vi "Autonomous Independent-NewMode.vi"() -> ()   [LabVIEW 2016]
doc: "This VI is called when autonomous begins, and will automatically be terminated when autonomous ends. You can carry out timed or sensor driven robot movement independently without needing to return to the caller."
uses:
  <vilib>/Rock Robotics/WPI/ThirdParty/CanMotor/TalonSRX/WPI_CANTalonSRX_BrakeOverride.ctl
  <vilib>/Rock Robotics/WPI/Utilities/WPI_GetSetVariantRefNum.vi
  <vilib>/Rock Robotics/Network Tables/NT Write Numeric Array.vi
  <vilib>/Rock Robotics/Network Tables/NT Read String.vi
  <vilib>/Rock Robotics/Network Tables/NT Read Numeric Array.vi
  <vilib>/Rock Robotics/Network Tables/NT Read String Array.vi
  Robot Global Data.vi
  <vilib>/Rock Robotics/WPI/RobotDrive/WPI_RobotDriveMecanumDrive_Cartesian.vi
  <vilib>/addons/control/pid/pid.llb/PID (DBL).vi
  <vilib>/Rock Robotics/Network Tables/NT Write String.vi
  <vilib>/Rock Robotics/Network Tables/NT Write Number.vi
  <vilib>/addons/control/pid/NI_PID_pid.lvlib
  ADIS16448-Teensy/ADIS16448-Teensy.lvlib
  <vilib>/ptbypt/NI_PtbyPt.lvlib
panel:
  out "VisionError":dbl
  out "RotateError":dbl
  in  "VisionIterationDelay":i32=100
  in  "VisionSampleLength":i32=10
  in  "RotateIterationDelay":i32=100
  in  "RotateSampleLength":i32=30
  in  "ExitLimitVision":dbl=0.2
  in  "ExitLimitRotate":dbl=0.1
  in  "Vision Align PID Gains":cluster{"Kp":dbl, "Ki":dbl, "Kd":dbl, "Kf":dbl}={"Kp"=0.006, "Ki"=1.6e-05, "Kd"=0.0, "Kf"=0.0002} {"Kf" format="%.6f"; "Kd" format="%.6f"; "Ki" format="%.6f"; "Kp" format="%.6f"}
  in  "Rotate PID gains":cluster{"Kp":dbl, "Ki":dbl, "Kd":dbl, "Kf":dbl}={"Kp"=0.0048, "Ki"=3e-05, "Kd"=0.02048, "Kf"=0.0} {"Kf" format="%.6f"; "Kd" format="%.6f"; "Ki" format="%.8f"; "Kp" format="%.6f"}
  out "Rotate Chart":cluster{dbl, "Z Angle":dbl}(graph)
  in  "Drive Slow PID Values":T1={"proportional gain (Kc)"=0.01, "integral time (Ti, min)"=0.0, "derivative time (Td, min)"=0.001}
  in  "Drive Slow Limits":cluster{"output high":dbl, "output low":dbl}={"output high"=0.25, "output low"=-0.25}
  out "Drive Slow":cluster{dbl, "Z Angle":dbl}(graph)
  in  "Strafe Correction":dbl=0.05 step=0.05 format="%#_13g"
  in  "Strafe PID Values":T1={"proportional gain (Kc)"=0.2, "integral time (Ti, min)"=0.0, "derivative time (Td, min)"=0.003} {"proportional gain (Kc)" step=0.01; "integral time (Ti, min)" step=0.001; "derivative time (Td, min)" step=0.001}
  in  "Strafe Angle Limits":cluster{"output high":dbl, "output low":dbl}={"output high"=0.1, "output low"=-0.1}
  out "Strafe Chart":cluster{dbl, "Z Angle":dbl}(graph)
  out "Drive Fast":cluster{dbl, "Z Angle":dbl}(graph)
  in  "Drive Fast Limits":cluster{"output high":dbl, "output low":dbl}={"output high"=0.25, "output low"=-0.25}
  in  "Rotate outputs":cluster{"output high":dbl, "output low":dbl}={"output high"=1.0, "output low"=-1.0} {"output high" step=0.1; "output low" step=0.1}
  out "Vision Align Rotate Chart":cluster{dbl, "Z Angle":dbl}(graph)
  in  "Vision Align Limits":cluster{"output high":dbl, "output low":dbl}={"output high"=1.0, "output low"=-1.0} {"output high" step=0.1; "output low" step=0.1}
  in  "Drive Fast PID Values":T1={"proportional gain (Kc)"=0.01, "integral time (Ti, min)"=0.0, "derivative time (Td, min)"=0.001}
  # "NEW MODE"
  # "Marvin:\n.025\n0\n.001"
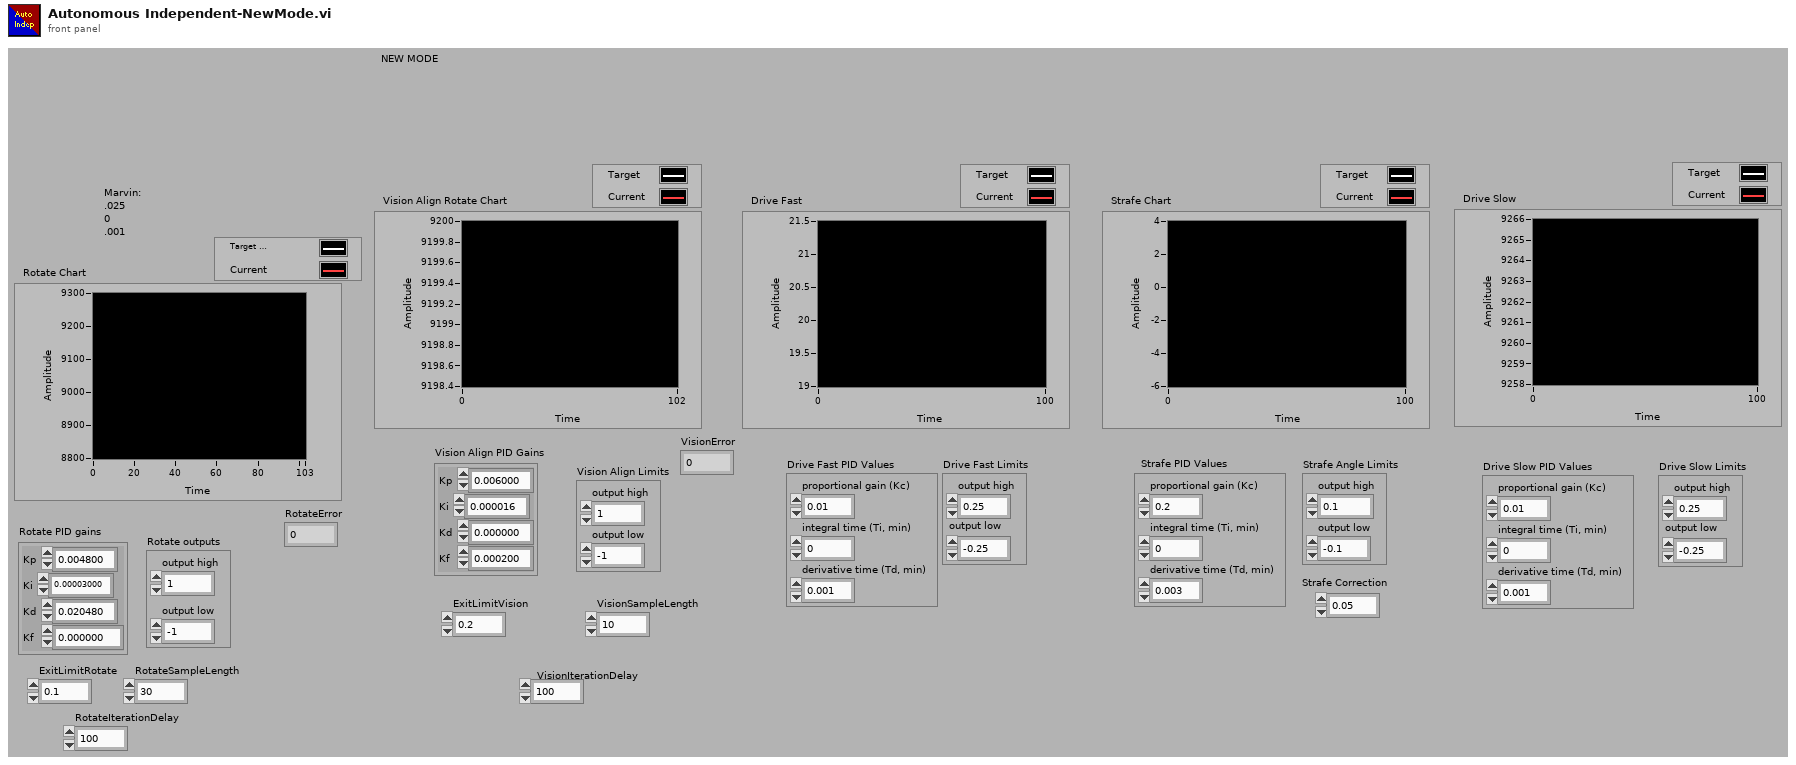
[diagram p1: front panel]
types:
  T1 = cluster{"proportional gain (Kc)":dbl, "integral time (Ti, min)":dbl, "derivative time (Td, min)":dbl}
  T2 = typedef "WPI_JoystickDevRef.ctl" = cluster{"Device":T3}
  T3 = typedef "WPI_JoystickDeviceEnum.ctl" = enum16{"USB 0", "USB 1", "USB 2", "USB 3", "USB 4", "USB 5"}
  T4 = typedef "WPI_CANTalonSRX_BrakeOverride.ctl" = enum8{"No Override", "Override to Coast", "Override to Brake"}
  T5 = typedef "WPI_MotorControlDeviceRef.ctl" = cluster{"DeviceStatus":errorcluster, "Type":T6, "PWM":cluster{"PWM Channel":T7, "DeadBand":T8}, "CAN":cluster{"Device Number":u8, "SetOutput VI Ref":variant, "GetOutput VI Ref":variant, "Enable VI Ref":variant, "Disable VI Ref":variant, "Data":variant}, "Invert":bool}
  T6 = typedef "WPI_MotorControlType.ctl" = enum16{"PWM", "CAN"}
  T7 = typedef "FPGA_DIOPWMChannel.ctl" = enum8{"PWM 0", "PWM 1", "PWM 2", "PWM 3", "PWM 4", "PWM 5", "PWM 6", "PWM 7", "PWM 8", "PWM 9", "PWM MXP 0", "PWM MXP 1", "PWM MXP 2", "PWM MXP 3", "PWM MXP 4", "PWM MXP 5", "PWM MXP 6", "PWM MXP 7", "PWM MXP 8", "PWM MXP 9", "Invalid"}
  T8 = typedef "WPI_PWMDeadband.ctl" = cluster{"Name":string, "maxPositivePwm":i32, "minPositivePwm":i32, "centerPwm":i32, "maxNegativePwm":i32, "minNegativePwm":i32, "angularRange":u16}
  T9 = typedef "WPI_SerialPortRef.ctl" = cluster{"DevStatus":errorcluster, "Serial Port Name":refnum<visa-resource-name>}
  T10 = typedef "WPI_RobotDriveDevRef.ctl" = cluster{"DevStatus":errorcluster, "Motors[]":T5[], "Square Inputs":bool, "Max Output":dbl}
  T11 = typedef "WPI_ServoDeviceRef.ctl" = cluster{"DeviceStatus":errorcluster, "PWM Channel":T7, "DeadBand":T8}
  T12 = cluster{"X Angle":dbl, "Y Angle":dbl, "Z Angle":dbl}
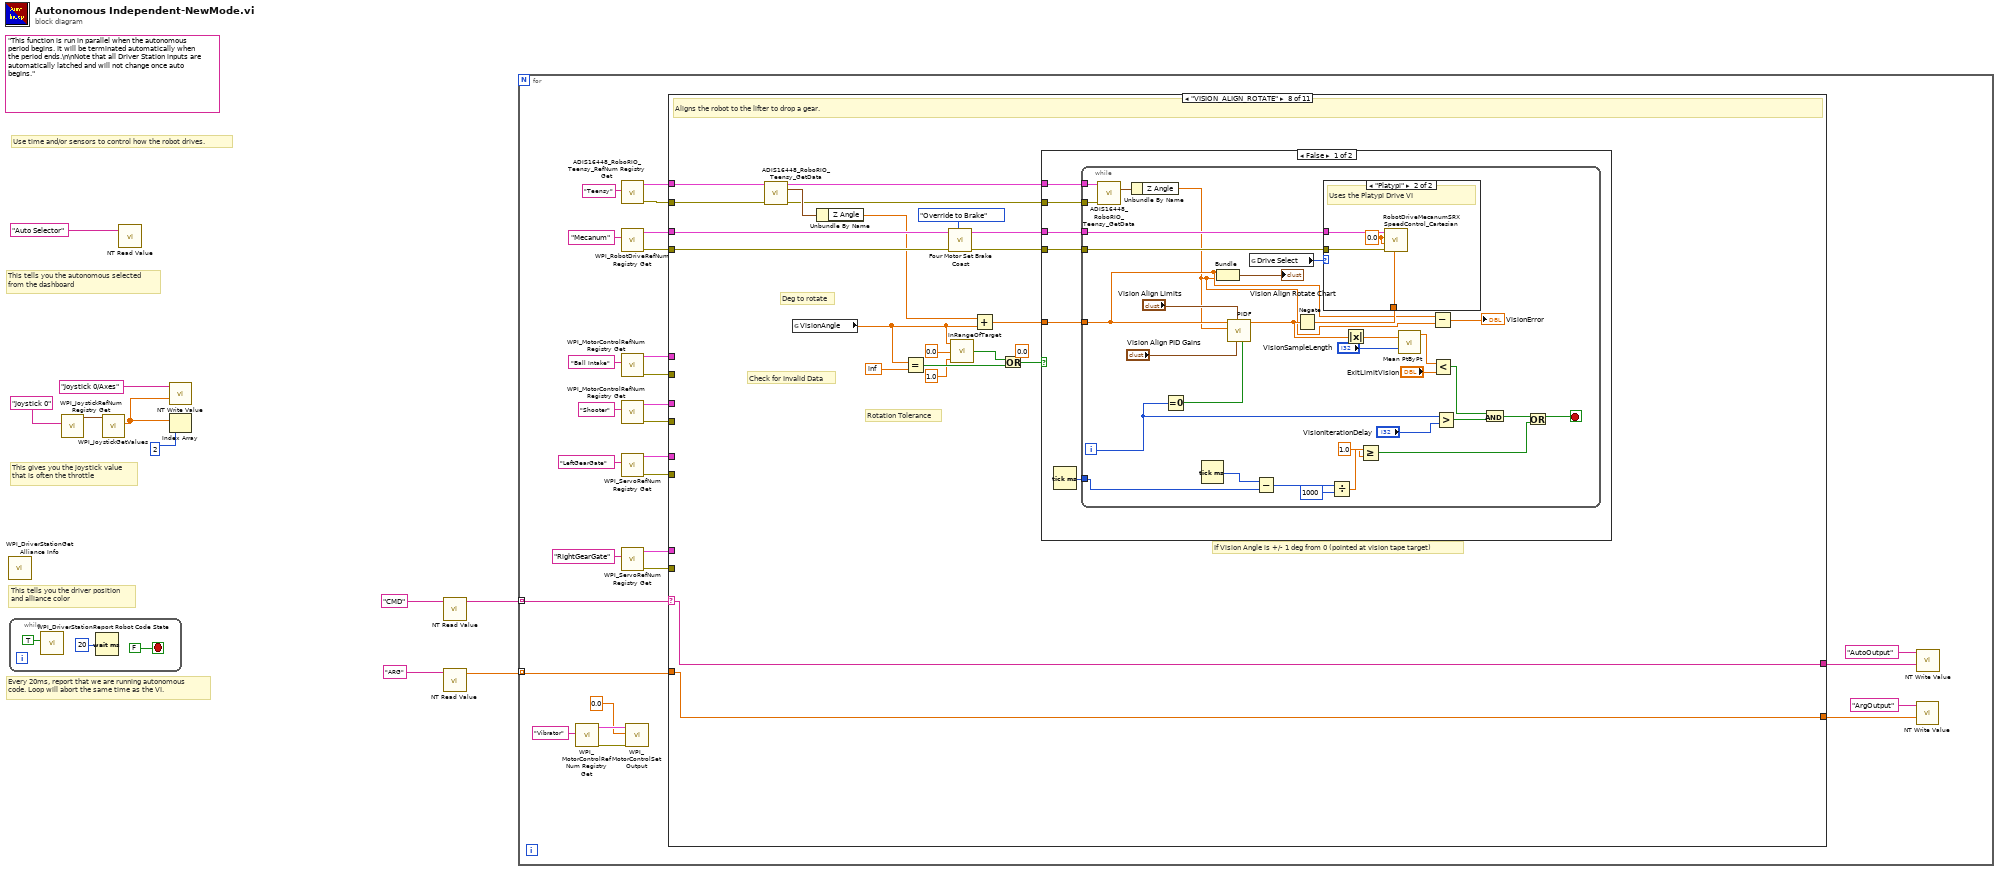
[diagram p0: block diagram]
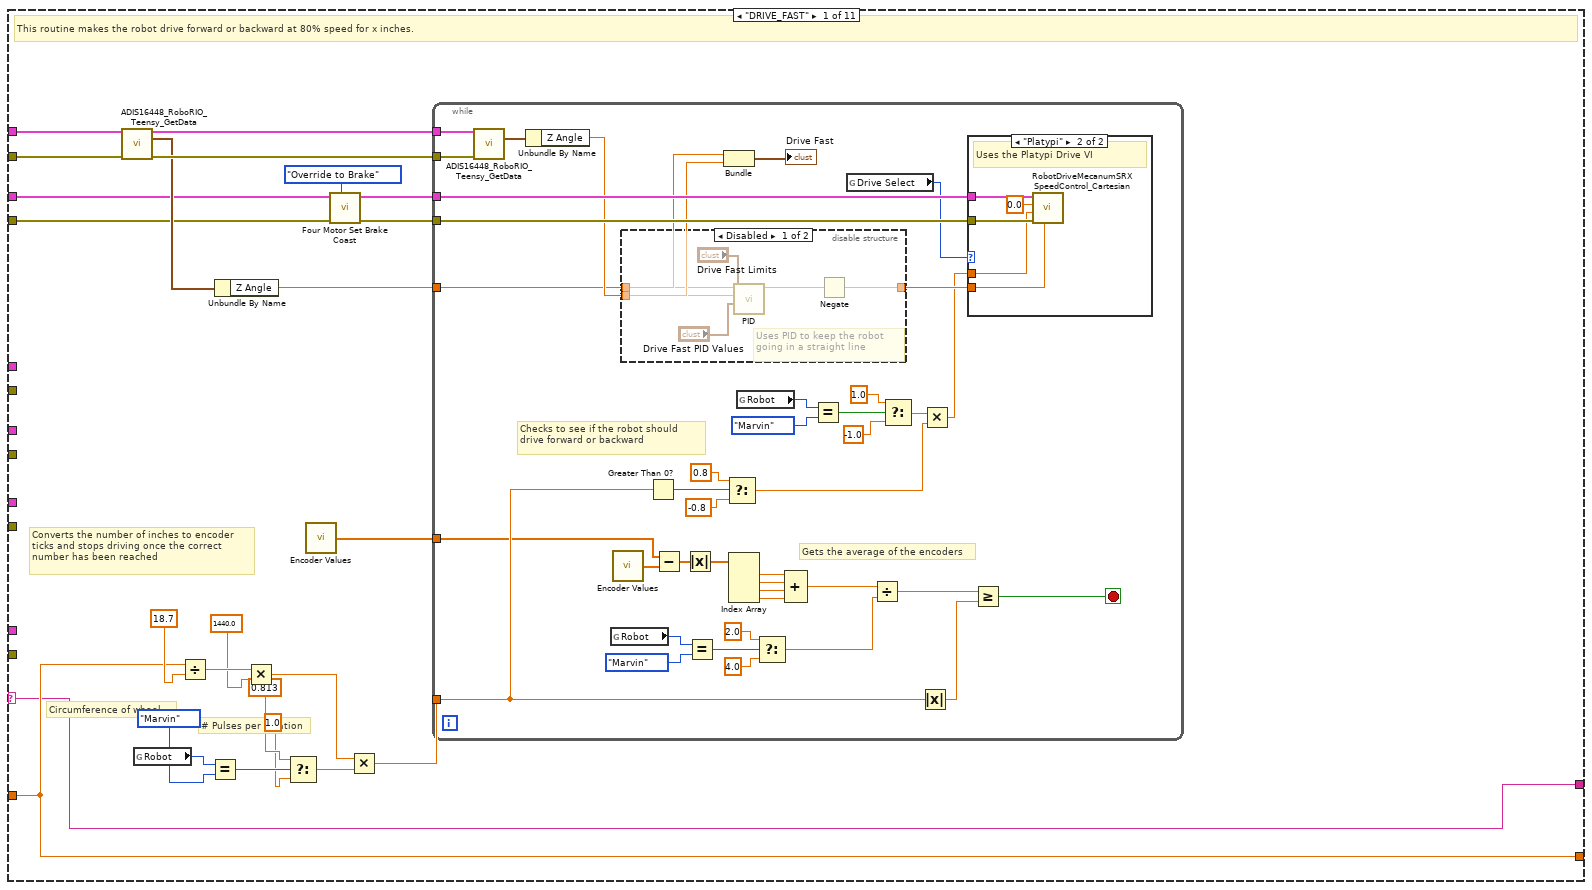
[diagram p2: hidden frame]
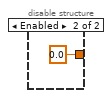
[diagram p3: hidden frame]
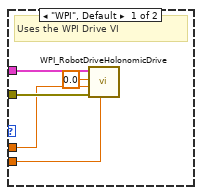
[diagram p4: hidden frame]
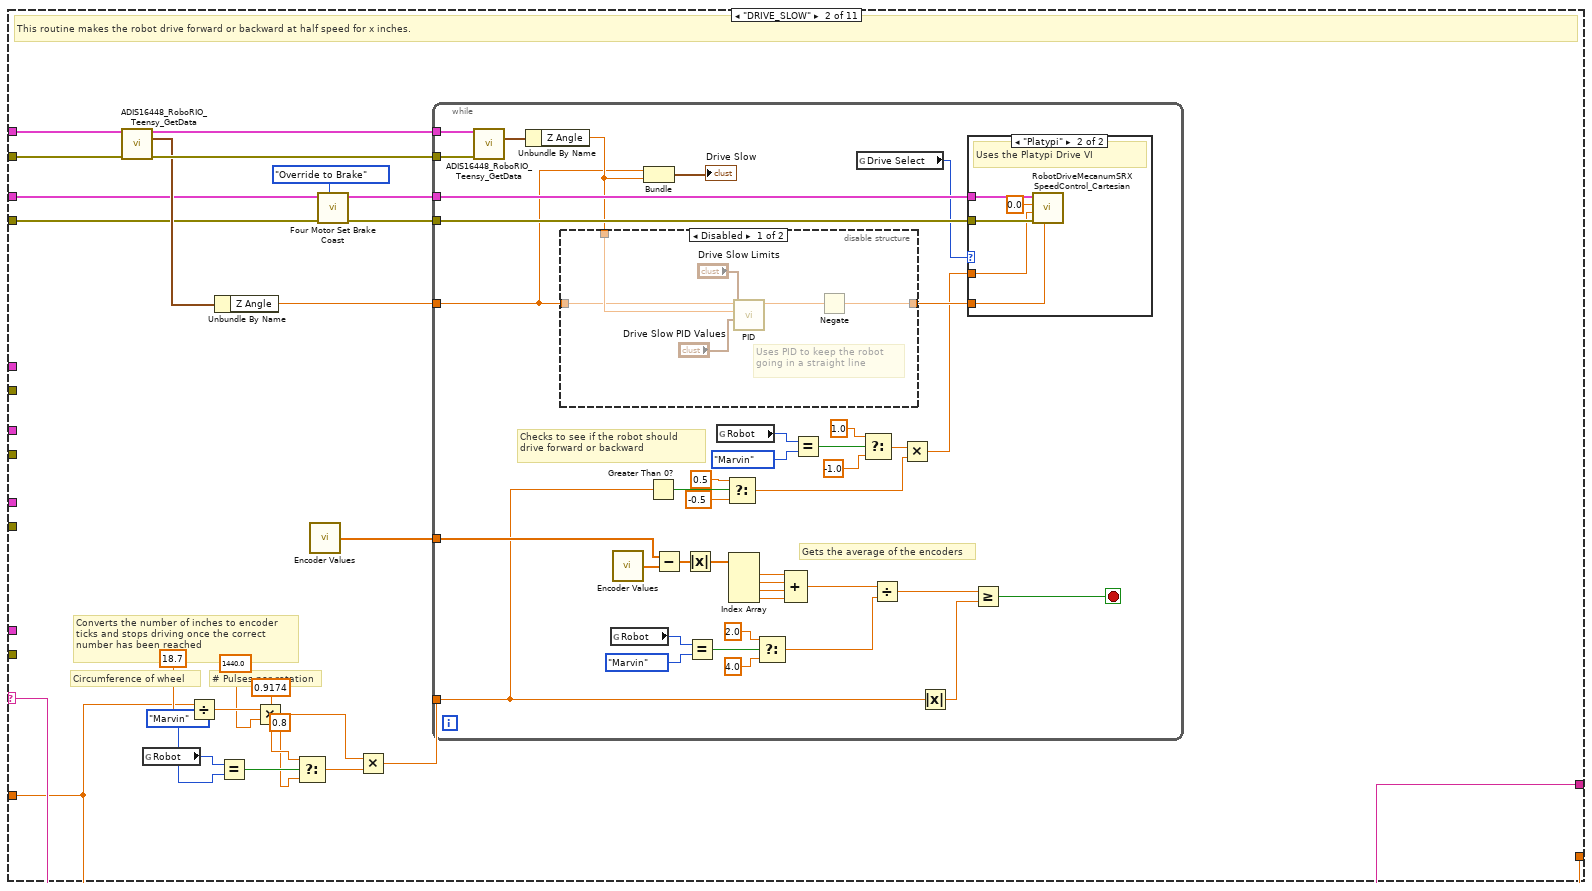
[diagram p5: hidden frame]
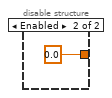
[diagram p6: hidden frame]
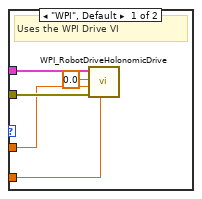
[diagram p7: hidden frame]
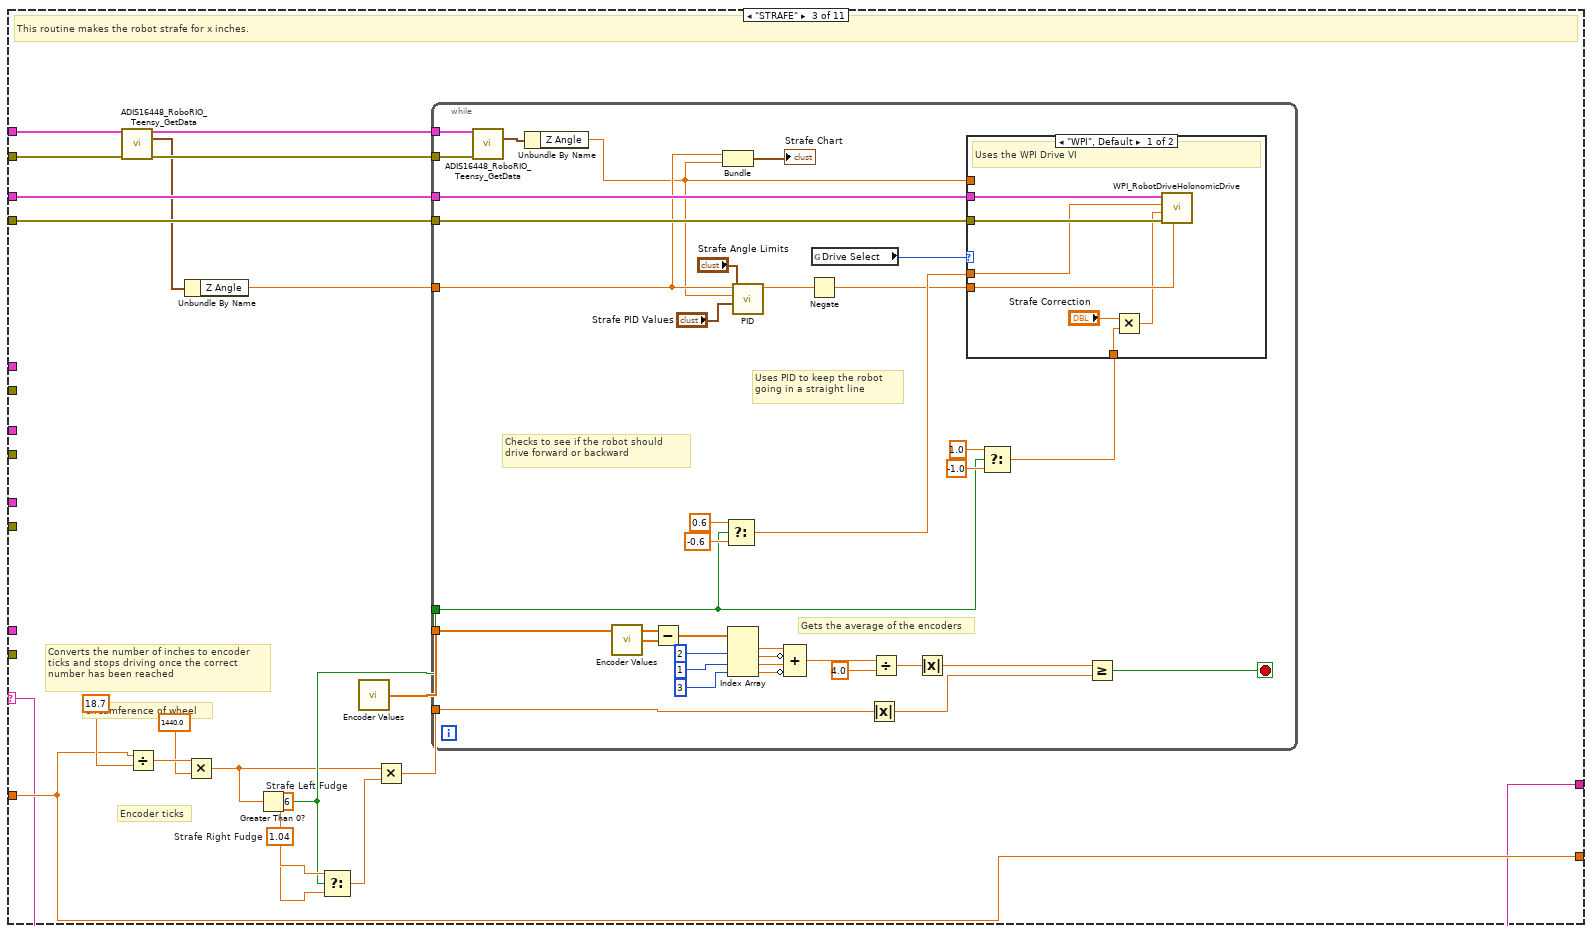
[diagram p8: hidden frame]
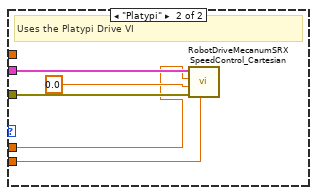
[diagram p9: hidden frame]
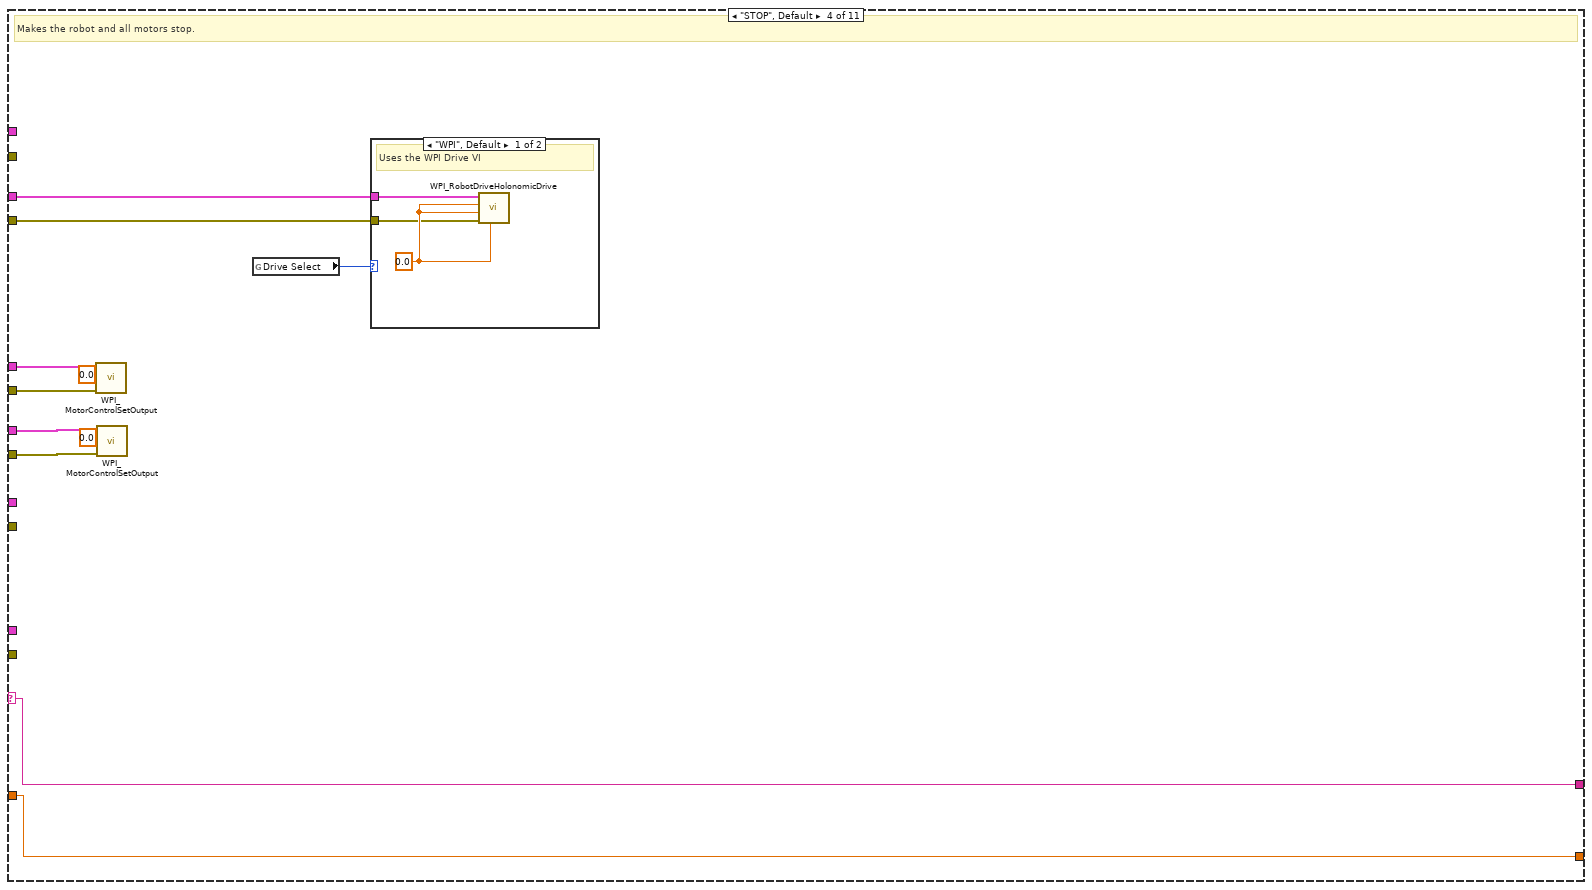
[diagram p10: hidden frame]
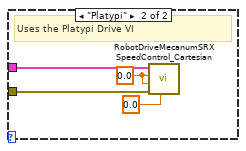
[diagram p11: hidden frame]
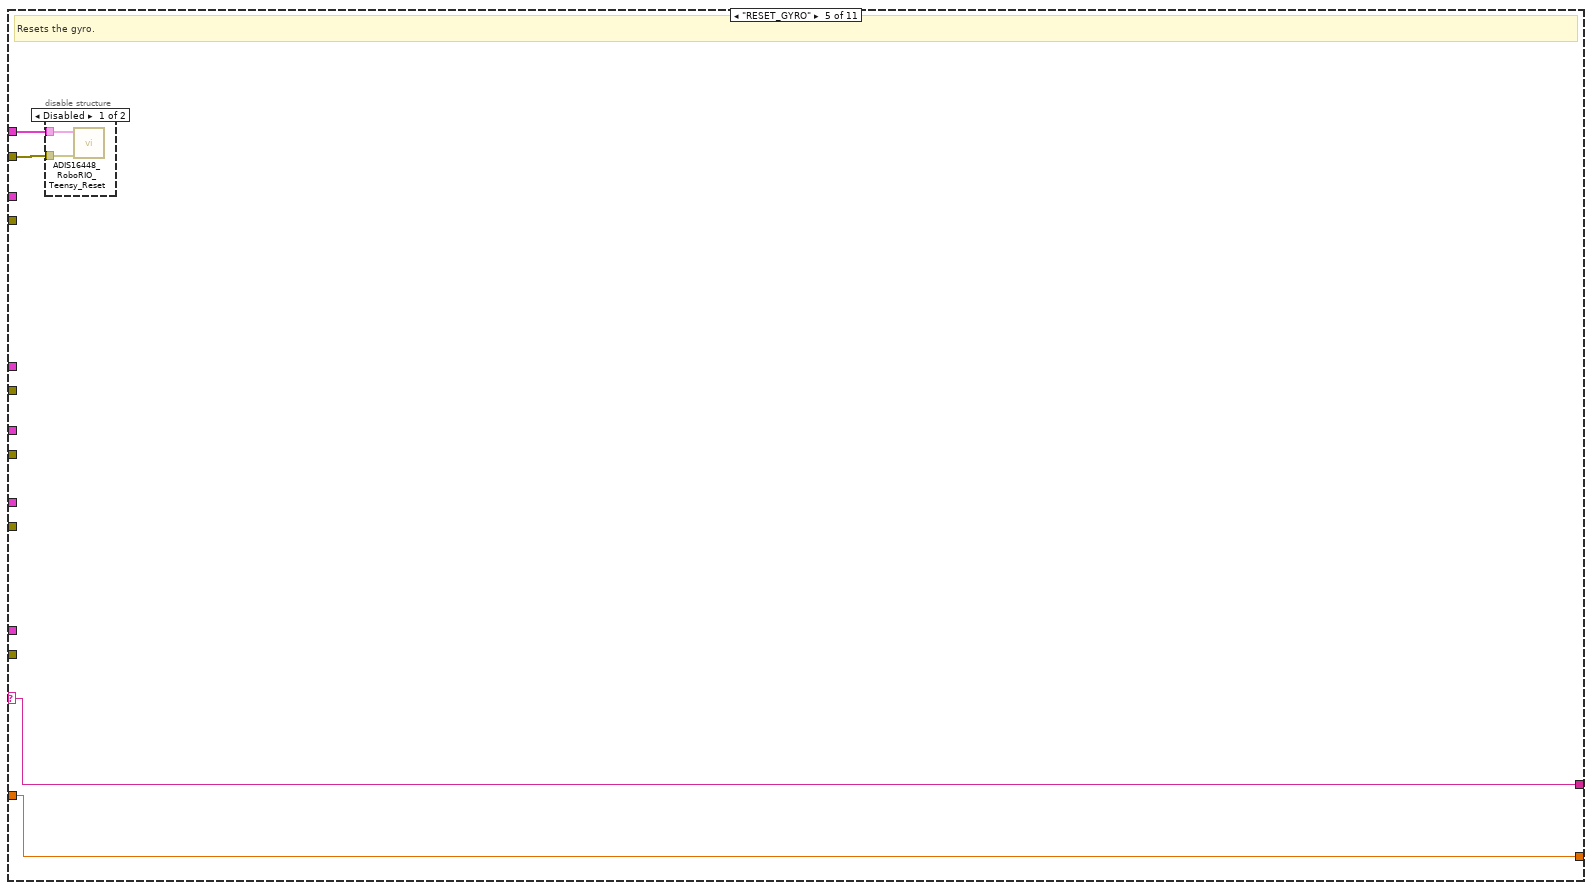
[diagram p12: hidden frame]
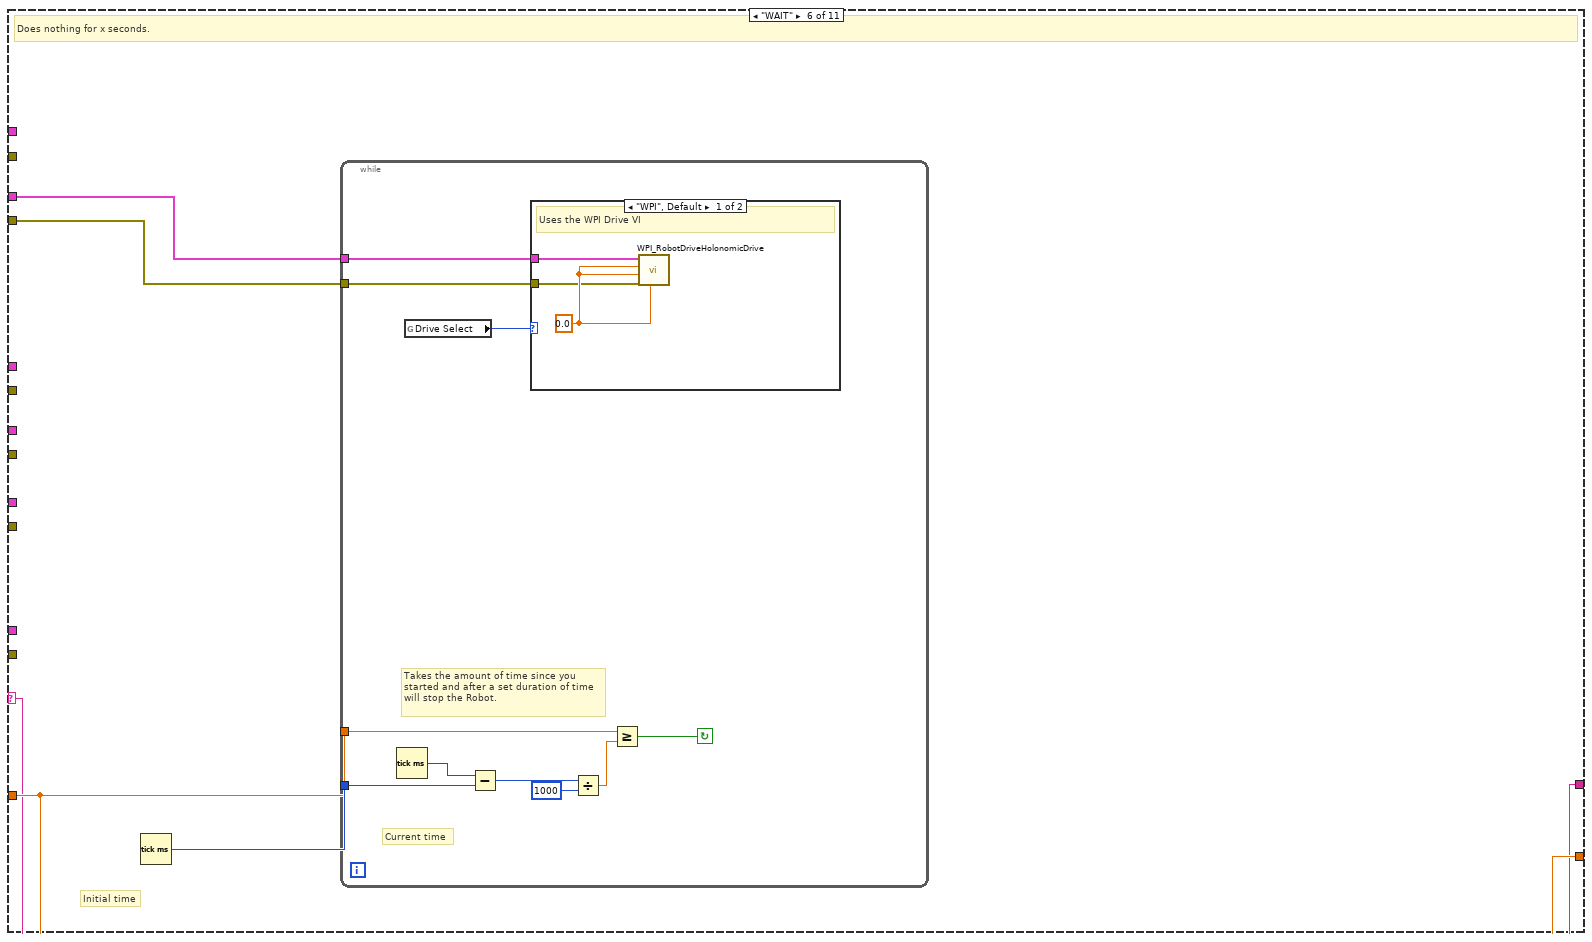
[diagram p14: hidden frame]
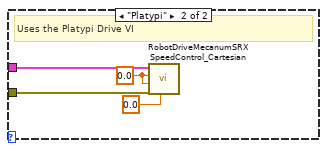
[diagram p15: hidden frame]
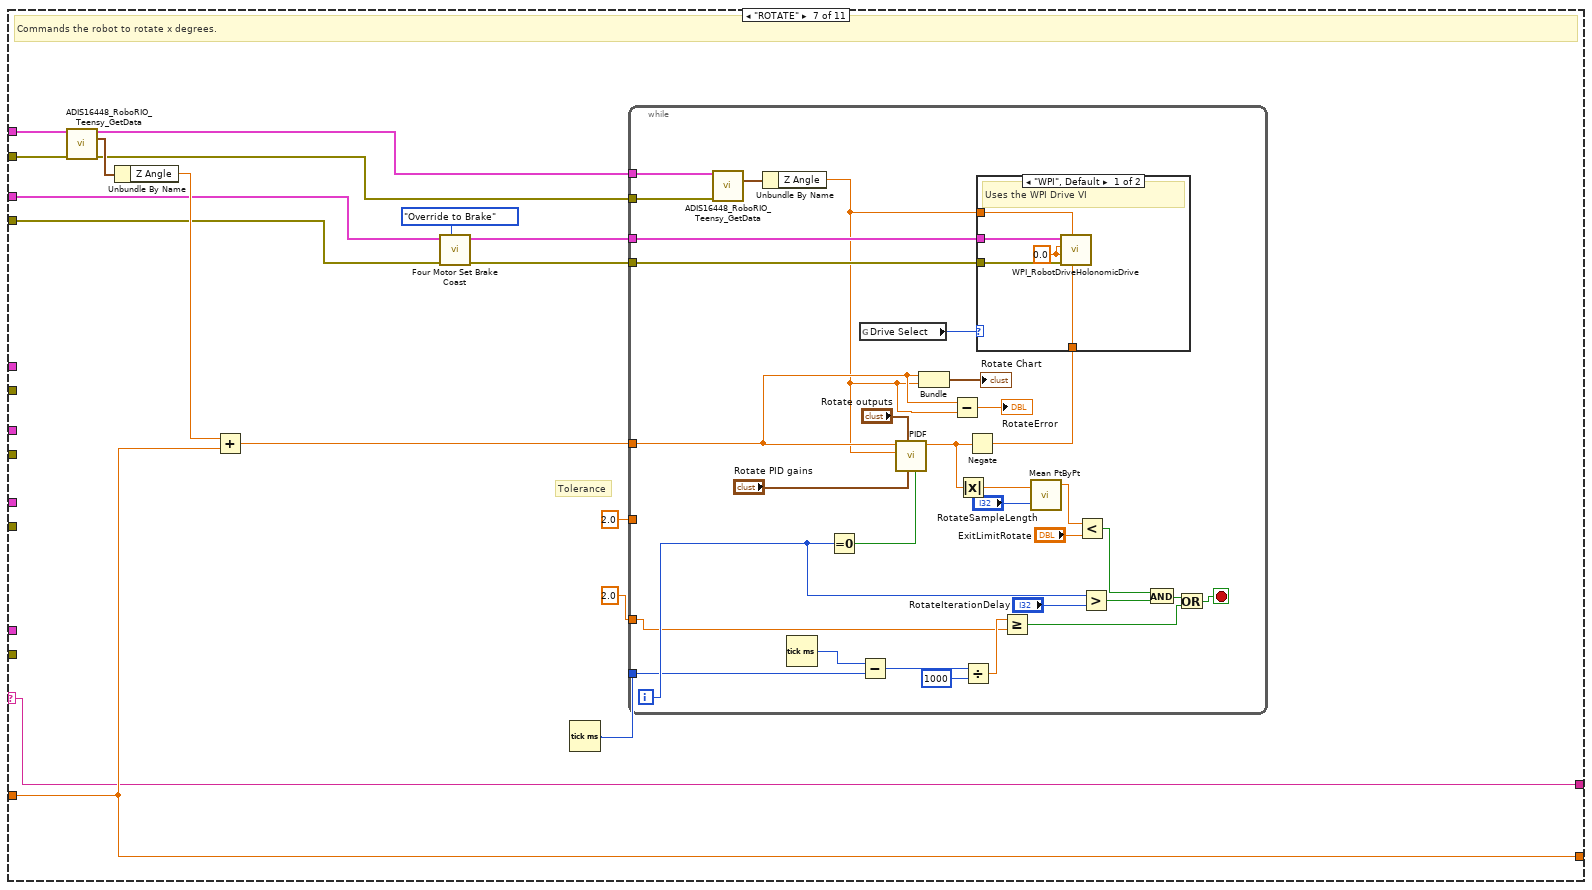
[diagram p16: hidden frame]
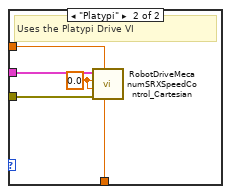
[diagram p17: hidden frame]
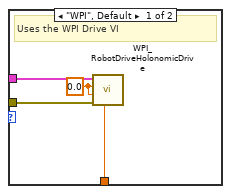
[diagram p18: hidden frame]
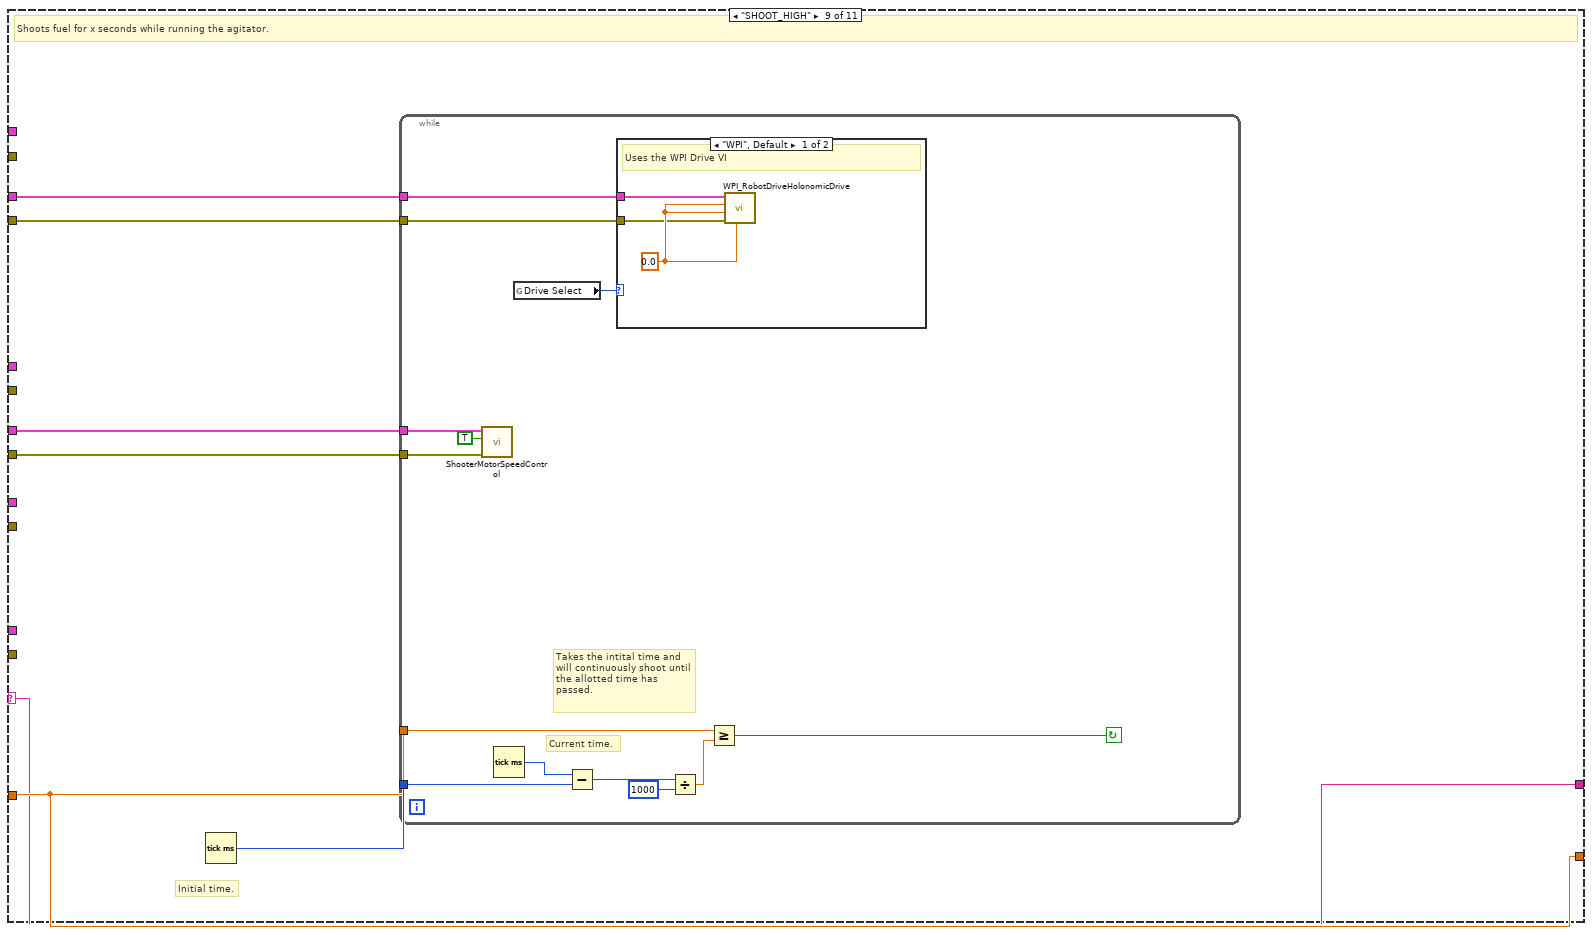
[diagram p20: hidden frame]
diagram:
  (unwired) "This function is run in parallel when the autonomous period begins. It will be terminated automatically when the period ends.\n\nNote that all Driver Station inputs are automatically latched and will not change once auto begins."
  # "Use time and/or sensors to control how the robot drives."
  # "This tells you the autonomous selected\nfrom the dashboard"
  # "Every 20ms, report that we are running autonomous\ncode. Loop will abort the same time as the VI."
  # "This gives you the joystick value\nthat is often the throttle"
  # "This tells you the driver position\nand alliance color"
  n1 = call <vilib>:"WPI_DriverStationGet Alliance Info.vi"() -> ()  [unwired: 12 out]
  n2 = while {
    stop <- FALSE stop-if-true
    n3 = call <vilib>:"WPI_DriverStationReport Robot Code State.vi"("Autonomous"=TRUE) -> ()  [unwired: 10 in, 1 out]
    n4 = Wait (ms)(milliseconds to wait=u32 20) -> ()  [unwired: 1 out]
  }
  n5 = call <vilib>:"WPI_JoystickRefNum Registry Get.vi"("refnum name"="Joystick 0") -> ("JoystickDevRef"=w9:T2)  [unwired: 1 in, 9 out]
  n6 = call <vilib>:"WPI_JoystickGetValues.vi"("JoystickDevRef"=w9) -> ("Axes"=w5:dbl[])  [unwired: 6 in, 4 out]
  n7 = call-poly <vilib>:"NT Read Value.vi"("Name"="Auto Selector") -> ()  [unwired: 9 in, 2 out]
  n8 = call-poly <vilib>:"NT Write Value.vi"("Numeric Array"=w5, "Name"="Joystick 0/Axes") -> ()  [unwired: 9 in, 1 out]
  n9 = Index Array(array=w5, index=u32 2 ("milliseconds to wait")) -> ()  [unwired: 1 out]
  n10 = call-poly <vilib>:"NT Read Value.vi"("Name"="ARG") -> ("Numeric Array"=w2:dbl[])  [unwired: 9 in, 1 out]
  n11 = call-poly <vilib>:"NT Read Value.vi"("Name"="CMD") -> ("String Array"=w1:string[])  [unwired: 9 in, 1 out]
  n12 = for {
    tunnel: w2 -> [w41] mode=indexing
    tunnel: w1 -> [w36] mode=indexing
    n13 = call <vilib>:"WPI_MotorControlRefNum Registry Get.vi"("refnum name"="Vibrator") -> ("error out"=w16:errorcluster, "MotorControlDevRef"=w15:T5)  [unwired: 9 in]
    n14 = call "ADIS16448_RoboRIO_Teensy_RefNum Registry Get.vi"("refnum name"="Teensy") -> ("error out"=w33:errorcluster, "SerialPortRefOut"=w34:T9)  [unwired: 9 in]
    n15 = call <vilib>:"WPI_RobotDriveRefNum Registry Get.vi"("refnum name"="Mecanum") -> ("error out"=w28:errorcluster, "RobotDriveDevRef"=w35:T10)  [unwired: 9 in]
    n16 = call <vilib>:"WPI_MotorControlRefNum Registry Get.vi"("refnum name"="Ball Intake") -> ("error out"=w31:errorcluster, "MotorControlDevRef"=w32:T5)  [unwired: 9 in]
    n17 = call <vilib>:"WPI_MotorControlRefNum Registry Get.vi"("refnum name"="Shooter") -> ("error out"=w29:errorcluster, "MotorControlDevRef"=w30:T5)  [unwired: 9 in]
    n18 = call <vilib>:"WPI_ServoRefNum Registry Get.vi"("refnum name"="LeftGearGate") -> ("error out"=w19:errorcluster, "ServoDeviceRef"=w20:T11)  [unwired: 9 in]
    n19 = call <vilib>:"WPI_ServoRefNum Registry Get.vi"("refnum name"="RightGearGate") -> ("error out"=w17:errorcluster, "ServoDeviceRef"=w18:T11)  [unwired: 9 in]
    n20 = call <vilib>:"WPI_MotorControlSetOutput.vi"("error in (no error)"=w16, "Output"=0.0, "MotorControlDevRef"=w15) -> ()  [unwired: 6 in, 3 out]
    n21 = case shown="\"VISION_ALIGN_ROTATE\"" w36 {
      selector: w36 -> [w49 w136 w204 w274 w291 w296 w320 w392 w444 w473 w481]
      tunnel: w41 -> [w50 w123 w205 w275 w290 w297 w321 w393 w445 w472 w480]
      tunnel: w35 -> [w52 w139 w222 w278 _ w299 w323 w395 w447 _ _]
      tunnel: w34 -> [w64 w145 w219 _ w292 _ w333 w397 _ _ _]
      tunnel: w33 -> [w65 w146 w221 _ w293 _ w332 w396 _ _ _]
      tunnel: w32 -> [_ _ _ w282 _ _ _ _ _ _ _]
      tunnel: w31 -> [_ _ _ w281 _ _ _ _ _ _ _]
      tunnel: w30 -> [_ _ _ w280 _ _ _ _ w449 _ _]
      tunnel: w29 -> [_ _ _ w279 _ _ _ _ w448 _ _]
      tunnel: w28 -> [w53 w138 w220 w277 _ w298 w324 w394 w446 _ _]
      tunnel: [w50 w123 w205 w275 w290 w297 w321 w393 w445 w472 w480] -> w24
      tunnel: [w49 w136 w204 w274 w291 w296 w320 w392 w444 w473 w481] -> w25
      tunnel: w20 -> [_ _ _ _ _ _ _ _ _ w477 w485]
      tunnel: w19 -> [_ _ _ _ _ _ _ _ _ w476 w484]
      tunnel: w18 -> [_ _ _ _ _ _ _ _ _ w475 w483]
      tunnel: w17 -> [_ _ _ _ _ _ _ _ _ w474 w482]
      frame "DRIVE_FAST" {
        # "# Pulses per rotation"
        # "Converts the number of inches to encoder ticks and stops driving once the correct number has been reached"
        # "Circumference of wheel"
        # "This routine makes the robot drive forward or backward at 80% speed for x inches."
        n22 = call "ADIS16448_RoboRIO_Teensy_GetData.vi"("SerialPortRefIn"=w64) -> ("SerialPortRefOut"=w63:T9, "IMU Angles Out"=w62:T12)  [unwired: 10 in, 3 out]
        n23 = global read "Robot Global Data.vi" "Robot"() -> (w47:enum16{"Unhinged", "Marvin"})
        n24 = Divide(x=w50, y=18.7) -> (x/y=w59:dbl)
        n25 = Equal?(x=w47, y=enum16{"Unhinged", "Marvin"}."Marvin") -> (x = y?=w46:bool)
        n26 = Unbundle By Name(w62) -> ("Z Angle"=w61:dbl)
        n27 = Multiply(x=w59, y=1440.0) -> (x*y=w56:dbl)
        n28 = Select(t=0.813, s=w46, f=1.0 ("Factor")) -> (s? t:f=w42:dbl)
        n29 = call "Encoder Values.vi"() -> ("Encoders"=w57:dbl[])  [unwired: 1 in]
        n30 = call "Four Motor Set Brake Coast.vi"("Brake / Coast Mode"=WPI_CANTalonSRX_BrakeOverride."Override to Brake", "error in (no error)"=w53, "RobotDriveDevRef in"=w52) -> ("error out"=w54:errorcluster, "RobotDriveDevRef out"=w55:T10)  [unwired: 7 in]
        n31 = Multiply(x=w56, y=w42) -> (x*y=w48:dbl)
        n32 = while {
          tunnel: w55 -> [w105]
          tunnel: w48 -> [w91]
          tunnel: w65 -> [w103]
          tunnel: w54 -> [w101]
          tunnel: w63 -> [w100]
          tunnel: w61 -> [w84]
          tunnel: w57 -> [w90]
          stop <- w104 stop-if-true
          # "Gets the average of the encoders"
          # "Checks to see if the robot should drive forward or backward"
          n33 = call "ADIS16448_RoboRIO_Teensy_GetData.vi"("SerialPortRefIn"=w100, "error in"=w103) -> ("IMU Angles Out"=w102:T12)  [unwired: 9 in, 4 out]
          n34 = Unbundle By Name(w102) -> ("Z Angle"=w85:dbl)
          n35 = global read "Robot Global Data.vi" "Robot"() -> (w80:enum16{"Unhinged", "Marvin"})
          n36 = call "Encoder Values.vi"() -> ("Encoders"=w89:dbl[])  [unwired: 1 in]
          n37 = disable-structure shown="Disabled" {
            disable-tunnel: w85 -> [w108 _]
            disable-tunnel: w84 -> [w107 _]
            disable-tunnel: [w106 0.0] -> w83
            frame Disabled {
              # "Uses PID to keep the robot going in a straight line"
              n38 = call-poly <vilib>:"PID.vi"("output range"="Drive Fast Limits", "PID gains"="Drive Fast PID Values", "process variable"=w108, "setpoint"=w107) -> ("output"=w109:dbl)  [unwired: 6 in, 1 out]
              n39 = Negate(x=w109) -> (-x=w106:dbl)
            }
            frame Enabled {
            }
          }
          n40 = Greater Than 0?(x=w91) -> (x > 0?=w99:bool)
          n41 = Subtract(x=w90, y=w89) -> (x-y=w88:dbl[])
          n42 = Absolute Value(x=w88) -> (abs(x)=w87:dbl[])
          n43 = Equal?(x=w80, y=enum16{"Unhinged", "Marvin"}."Marvin") -> (x = y?=w79:bool)
          n44 = Bundle("Z Angle"=w84, "Z Angle"=w85) -> (→"Drive Fast":cluster{"Z Angle":dbl, "Z Angle":dbl})  [unwired: 1 in]
          n45 = Select(t=0.8, s=w99, f=-0.8) -> (s? t:f=w67:dbl)
          n46 = Index Array(array=w87) -> (element #1=w95:dbl, element #2=w93:dbl, element #3=w92:dbl, element #4=w94:dbl)  [unwired: 4 in]
          n47 = global read "Robot Global Data.vi" "Robot"() -> (w73:enum16{"Unhinged", "Marvin"})
          n48 = Select(t=2.0, s=w79, f=4.0) -> (s? t:f=w76:dbl)
          n49 = Compound Arithmetic op=ADD(w95, w93, w92, w94) -> (w96:dbl)
          n50 = Equal?(x=w73, y=enum16{"Unhinged", "Marvin"}."Marvin") -> (x = y?=w72:bool)
          n51 = global read "Robot Global Data.vi" "Drive Select"() -> (w74:enum16{"WPI", "Platypi"})
          n52 = Divide(x=w96, y=w76) -> (x/y=w81:dbl)
          n53 = Select(t=1.0, s=w72, f=-1.0 ("Factor")) -> (s? t:f=w68:dbl)
          n54 = Absolute Value(x=w91) -> (abs(x)=w82:dbl)
          n55 = Multiply(x=w68, y=w67) -> (x*y=w69:dbl)
          n56 = case shown="\"Platypi\"" w74 {
            tunnel: w105 -> [w117 w122]
            tunnel: w101 -> [w115 w121]
            tunnel: w83 -> [w114 w119]
            tunnel: w69 -> [w113 w118]
            frame "WPI", Default {
              # "Uses the WPI Drive VI"
              n57 = call-poly <vilib>:"WPI_RobotDriveHolonomicDrive.vi"("Rotation"=w114, "error in (no error)"=w115, "Y"=w113, "X"=0.0, "RobotDriveDevRef"=w117) -> ()  [unwired: 4 in, 3 out]
            }
            frame "Platypi" {
              # "Uses the Platypi Drive VI"
              n58 = call "RobotDriveMecanumSRXSpeedControl_Cartesian.vi"("Rotation"=w119, "error in (no error)"=w121, "Y"=w118, "X"=0.0, "RobotDriveDevRef"=w122) -> ()  [unwired: 3 in, 4 out]
            }
          }
          n59 = Greater Or Equal?(x=w81, y=w82) -> (x >= y?=w104:bool)
        }
      }
      frame "DRIVE_SLOW" {
        # "# Pulses per rotation"
        # "Circumference of wheel"
        # "Converts the number of inches to encoder ticks and stops driving once the correct number has been reached"
        # "This routine makes the robot drive forward or backward at half speed for x inches."
        n60 = call "ADIS16448_RoboRIO_Teensy_GetData.vi"("SerialPortRefIn"=w145) -> ("SerialPortRefOut"=w144:T9, "IMU Angles Out"=w143:T12)  [unwired: 10 in, 3 out]
        n61 = global read "Robot Global Data.vi" "Robot"() -> (w130:enum16{"Unhinged", "Marvin"})
        n62 = Divide(x=w123, y=18.7) -> (x/y=w133:dbl)
        n63 = Unbundle By Name(w143) -> ("Z Angle"=w142:dbl)
        n64 = Equal?(x=w130, y=enum16{"Unhinged", "Marvin"}."Marvin") -> (x = y?=w129:bool)
        n65 = Multiply(x=w133, y=1440.0) -> (x*y=w131:dbl)
        n66 = Select(t=0.9174, s=w129, f=0.8 ("Factor")) -> (s? t:f=w125:dbl)
        n67 = call "Encoder Values.vi"() -> ("Encoders"=w135:dbl[])  [unwired: 1 in]
        n68 = call "Four Motor Set Brake Coast.vi"("Brake / Coast Mode"=WPI_CANTalonSRX_BrakeOverride."Override to Brake", "error in (no error)"=w138, "RobotDriveDevRef in"=w139) -> ("error out"=w140:errorcluster, "RobotDriveDevRef out"=w141:T10)  [unwired: 7 in]
        n69 = Multiply(x=w131, y=w125) -> (x*y=w124:dbl)
        n70 = while {
          tunnel: w141 -> [w186]
          tunnel: w146 -> [w185]
          tunnel: w140 -> [w183]
          tunnel: w144 -> [w182]
          tunnel: w142 -> [w176]
          tunnel: w135 -> [w158]
          tunnel: w124 -> [w157]
          stop <- w156 stop-if-true
          # "Gets the average of the encoders"
          # "Checks to see if the robot should drive forward or backward"
          n71 = call "ADIS16448_RoboRIO_Teensy_GetData.vi"("SerialPortRefIn"=w182, "error in"=w185) -> ("IMU Angles Out"=w184:T12)  [unwired: 9 in, 4 out]
          n72 = Unbundle By Name(w184) -> ("Z Angle"=w177:dbl)
          n73 = disable-structure shown="Disabled" {
            disable-tunnel: w177 -> [w189 _]
            disable-tunnel: w176 -> [w188 _]
            disable-tunnel: [w187 0.0] -> w175
            frame Disabled {
              # "Uses PID to keep the robot going in a straight line"
              n74 = call-poly <vilib>:"PID.vi"("output range"="Drive Slow Limits", "PID gains"="Drive Slow PID Values", "process variable"=w189, "setpoint"=w188) -> ("output"=w190:dbl)  [unwired: 6 in, 1 out]
              n75 = Negate(x=w190) -> (-x=w187:dbl)
            }
            frame Enabled {
            }
          }
          n76 = global read "Robot Global Data.vi" "Robot"() -> (w164:enum16{"Unhinged", "Marvin"})
          n77 = call "Encoder Values.vi"() -> ("Encoders"=w169:dbl[])  [unwired: 1 in]
          n78 = Bundle("Z Angle"=w176, "Z Angle"=w177) -> (→"Drive Slow":cluster{"Z Angle":dbl, "Z Angle":dbl})  [unwired: 1 in]
          n79 = Greater Than 0?(x=w157) -> (x > 0?=w181:bool)
          n80 = Subtract(x=w158, y=w169) -> (x-y=w168:dbl[])
          n81 = Absolute Value(x=w168) -> (abs(x)=w167:dbl[])
          n82 = Equal?(x=w164, y=enum16{"Unhinged", "Marvin"}."Marvin") -> (x = y?=w163:bool)
          n83 = global read "Robot Global Data.vi" "Robot"() -> (w154:enum16{"Unhinged", "Marvin"})
          n84 = Select(t=0.5, s=w181, f=-0.5) -> (s? t:f=w147:dbl)
          n85 = Index Array(array=w167) -> (element #1=w173:dbl, element #2=w171:dbl, element #3=w170:dbl, element #4=w172:dbl)  [unwired: 4 in]
          n86 = Select(t=2.0, s=w163, f=4.0) -> (s? t:f=w160:dbl)
          n87 = Compound Arithmetic op=ADD(w173, w171, w170, w172) -> (w174:dbl)
          n88 = Equal?(x=w154, y=enum16{"Unhinged", "Marvin"}."Marvin") -> (x = y?=w153:bool)
          n89 = global read "Robot Global Data.vi" "Drive Select"() -> (w155:enum16{"WPI", "Platypi"})
          n90 = Select(t=1.0, s=w153, f=-1.0 ("Factor")) -> (s? t:f=w151:dbl)
          n91 = Divide(x=w174, y=w160) -> (x/y=w165:dbl)
          n92 = Multiply(x=w151, y=w147) -> (x*y=w150:dbl)
          n93 = Absolute Value(x=w157) -> (abs(x)=w166:dbl)
          n94 = case shown="\"Platypi\"" w155 {
            tunnel: w186 -> [w198 w203]
            tunnel: w183 -> [w196 w202]
            tunnel: w175 -> [w195 w200]
            tunnel: w150 -> [w194 w199]
            frame "WPI", Default {
              # "Uses the WPI Drive VI"
              n95 = call-poly <vilib>:"WPI_RobotDriveHolonomicDrive.vi"("Rotation"=w195, "error in (no error)"=w196, "Y"=w194, "X"=0.0, "RobotDriveDevRef"=w198) -> ()  [unwired: 4 in, 3 out]
            }
            frame "Platypi" {
              # "Uses the Platypi Drive VI"
              n96 = call "RobotDriveMecanumSRXSpeedControl_Cartesian.vi"("Rotation"=w200, "error in (no error)"=w202, "Y"=w199, "X"=0.0, "RobotDriveDevRef"=w203) -> ()  [unwired: 3 in, 4 out]
            }
          }
          n97 = Greater Or Equal?(x=w165, y=w166) -> (x >= y?=w156:bool)
        }
      }
      frame "STRAFE" {
        w209 = 1.04  # Strafe Right Fudge
        w210 = 1.16  # Strafe Left Fudge
        # "Converts the number of inches to encoder ticks and stops driving once the correct number has been reached"
        # "Circumference of wheel"
        # "Encoder ticks"
        # "This routine makes the robot strafe for x inches."
        n98 = call "ADIS16448_RoboRIO_Teensy_GetData.vi"("SerialPortRefIn"=w219) -> ("SerialPortRefOut"=w218:T9, "IMU Angles Out"=w217:T12)  [unwired: 10 in, 3 out]
        n99 = Divide(x=w205, y=18.7) -> (x/y=w214:dbl)
        n100 = Unbundle By Name(w217) -> ("Z Angle"=w216:dbl)
        n101 = Multiply(x=w214, y=1440.0) -> (x*y=w206:dbl)
        n102 = Greater Than 0?(x=w206) -> (x > 0?=w207:bool)
        n103 = Select(t=w210, s=w207, f=w209) -> (s? t:f=w208:dbl)
        n104 = call "Encoder Values.vi"() -> ("Encoders"=w212:dbl[])  [unwired: 1 in]
        n105 = Multiply(x=w206, y=w208) -> (x*y=w211:dbl)
        n106 = while {
          tunnel: w222 -> [w259]
          tunnel: w211 -> [w239]
          tunnel: w221 -> [w254]
          tunnel: w220 -> [w252]
          tunnel: w218 -> [w249]
          tunnel: w216 -> [w235]
          tunnel: w212 -> [w238]
          tunnel: w207 -> [w223]
          stop <- w255 stop-if-true
          # "Gets the average of the encoders"
          # "Uses PID to keep the robot going in a straight line"
          # "Checks to see if the robot should drive forward or backward"
          n107 = call "ADIS16448_RoboRIO_Teensy_GetData.vi"("SerialPortRefIn"=w249, "error in"=w254) -> ("IMU Angles Out"=w253:T12)  [unwired: 9 in, 4 out]
          n108 = Unbundle By Name(w253) -> ("Z Angle"=w232:dbl)
          n109 = call "Encoder Values.vi"() -> ("Encoders"=w237:dbl[])  [unwired: 1 in]
          n110 = Subtract(x=w238, y=w237) -> (x-y=w227:dbl[])
          n111 = Bundle("Z Angle"=w235, "Z Angle"=w232) -> (→"Strafe Chart":cluster{"Z Angle":dbl, "Z Angle":dbl})  [unwired: 1 in]
          n112 = Select(t=0.6, s=w223, f=-0.6) -> (s? t:f=w240:dbl)
          n113 = Index Array(array=w227, index #1=2 ("index"), index #3=1 ("index"), index #4=3 ("index")) -> (element #1=w244:dbl, element #2=w242:dbl, element #3=w241:dbl, element #4=w243:dbl)  [unwired: 1 in]
          n114 = call-poly <vilib>:"PID.vi"("output range"="Strafe Angle Limits", "PID gains"="Strafe PID Values", "process variable"=w232, "setpoint"=w235) -> ("output"=w234:dbl)  [unwired: 6 in, 1 out]
          n115 = Compound Arithmetic op=ADD(w244, invert w242, w241, invert w243) -> (w245:dbl)
          n116 = Negate(x=w234) -> (-x=w233:dbl)
          n117 = global read "Robot Global Data.vi" "Drive Select"() -> (w250:enum16{"WPI", "Platypi"})
          n118 = Absolute Value(x=w239) -> (abs(x)=w228:dbl)
          n119 = Divide(x=w245, y=4.0) -> (x/y=w257:dbl)
          n120 = Absolute Value(x=w257) -> (abs(x)=w256:dbl)
          n121 = Select(t=1.0, s=w223, f=-1.0) -> (s? t:f=w224:dbl)
          n122 = case shown="\"WPI\", Default" w250 {
            tunnel: w259 -> [w266 w271]
            tunnel: w252 -> [w265 w270]
            tunnel: w233 -> [w264 w269]
            tunnel: w240 -> [w263 w267]
            tunnel: w232 -> [_ _]
            tunnel: w224 -> [w260 _]
            frame "WPI", Default {
              # "Uses the WPI Drive VI"
              n123 = Multiply(x="Strafe Correction", y=w260) -> (x*y=w261:dbl)
              n124 = call-poly <vilib>:"WPI_RobotDriveHolonomicDrive.vi"("Rotation"=w264, "error in (no error)"=w265, "Y"=w261, "X"=w263, "RobotDriveDevRef"=w266) -> ()  [unwired: 4 in, 3 out]
            }
            frame "Platypi" {
              # "Uses the Platypi Drive VI"
              n125 = call "RobotDriveMecanumSRXSpeedControl_Cartesian.vi"("Rotation"=w269, "error in (no error)"=w270, "Y"=0.0 ("X"), "X"=w267, "RobotDriveDevRef"=w271) -> ()  [unwired: 3 in, 4 out]
            }
          }
          n126 = Greater Or Equal?(x=w256, y=w228) -> (x >= y?=w255:bool)
        }
      }
      frame "STOP", Default {
        # "Makes the robot and all motors stop."
        n127 = call <vilib>:"WPI_MotorControlSetOutput.vi"("error in (no error)"=w281, "Output"=0.0, "MotorControlDevRef"=w282) -> ()  [unwired: 6 in, 3 out]
        n128 = call <vilib>:"WPI_MotorControlSetOutput.vi"("error in (no error)"=w279, "Output"=0.0, "MotorControlDevRef"=w280) -> ()  [unwired: 6 in, 3 out]
        n129 = global read "Robot Global Data.vi" "Drive Select"() -> (w276:enum16{"WPI", "Platypi"})
        n130 = case shown="\"WPI\", Default" w276 {
          tunnel: w278 -> [w283 w289]
          tunnel: w277 -> [w284 w288]
          frame "WPI", Default {
            w285 = 0.0 ("Y")
            # "Uses the WPI Drive VI"
            n131 = call-poly <vilib>:"WPI_RobotDriveHolonomicDrive.vi"("Rotation"=w285, "error in (no error)"=w284, "Y"=w285, "X"=w285, "RobotDriveDevRef"=w283) -> ()  [unwired: 4 in, 3 out]
          }
          frame "Platypi" {
            w287 = 0.0 ("X")
            # "Uses the Platypi Drive VI"
            n132 = call "RobotDriveMecanumSRXSpeedControl_Cartesian.vi"("Rotation"=0.0, "error in (no error)"=w288, "Y"=w287, "X"=w287, "RobotDriveDevRef"=w289) -> ()  [unwired: 3 in, 4 out]
          }
        }
      }
      frame "RESET_GYRO" {
        # "Resets the gyro."
        n133 = disable-structure shown="Disabled" {
          disable-tunnel: w293 -> [w295 _]
          disable-tunnel: w292 -> [w294 _]
          frame Disabled {
            n134 = call "ADIS16448_RoboRIO_Teensy_Reset.vi"("error in"=w295, "SerialPortRef"=w294) -> ()  [unwired: 8 in, 2 out]
          }
          frame Enabled {
          }
        }
      }
      frame "WAIT" {
        # "Initial time"
        # "Does nothing for x seconds."
        n135 = Tick Count (ms)() -> (millisecond timer value=w300:u32)
        n136 = while {
          tunnel: w297 -> [w305]
          tunnel: w300 -> [w310]
          tunnel: w299 -> [w303]
          tunnel: w298 -> [w302]
          stop <- w304 continue-if-true
          # "Current time"
          # "Takes the amount of time since you started and after a set duration of time will stop the Robot."
          n137 = Tick Count (ms)() -> (millisecond timer value=w309:u32)
          n138 = global read "Robot Global Data.vi" "Drive Select"() -> (w301:enum16{"WPI", "Platypi"})
          n139 = Subtract(x=w309, y=w310) -> (x-y=w308:u32)
          n140 = case shown="\"WPI\", Default" w301 {
            tunnel: w303 -> [w311 w317]
            tunnel: w302 -> [w312 w316]
            frame "WPI", Default {
              w313 = 0.0 ("Y")
              # "Uses the WPI Drive VI"
              n141 = call-poly <vilib>:"WPI_RobotDriveHolonomicDrive.vi"("Rotation"=w313, "error in (no error)"=w312, "Y"=w313, "X"=w313, "RobotDriveDevRef"=w311) -> ()  [unwired: 4 in, 3 out]
            }
            frame "Platypi" {
              w315 = 0.0 ("X")
              # "Uses the Platypi Drive VI"
              n142 = call "RobotDriveMecanumSRXSpeedControl_Cartesian.vi"("Rotation"=0.0, "error in (no error)"=w316, "Y"=w315, "X"=w315, "RobotDriveDevRef"=w317) -> ()  [unwired: 3 in, 4 out]
            }
          }
          n143 = Divide(x=w308, y=u32 1000) -> (x/y=w306:dbl)
          n144 = Greater Or Equal?(x=w305, y=w306) -> (x >= y?=w304:bool)
        }
      }
      frame "ROTATE" {
        # "Tolerance"
        # "Commands the robot to rotate x degrees."
        n145 = call "ADIS16448_RoboRIO_Teensy_GetData.vi"("SerialPortRefIn"=w333, "error in"=w332) -> ("SerialPortRefOut"=w331:T9, "IMU Angles Out"=w334:T12, "error out"=w330:errorcluster)  [unwired: 9 in, 2 out]
        n146 = Unbundle By Name(w334) -> ("Z Angle"=w329:dbl)
        n147 = Add(x=w329, y=w321) -> (x+y=w328:dbl)
        n148 = call "Four Motor Set Brake Coast.vi"("Brake / Coast Mode"=WPI_CANTalonSRX_BrakeOverride."Override to Brake", "error in (no error)"=w324, "RobotDriveDevRef in"=w323) -> ("error out"=w325:errorcluster, "RobotDriveDevRef out"=w326:T10)  [unwired: 7 in]
        n149 = Tick Count (ms)() -> (millisecond timer value=w319:u32)
        n150 = while {
          tunnel: w331 -> [w362]
          tunnel: w330 -> [w366]
          tunnel: w328 -> [w346]
          tunnel: w326 -> [w364]
          tunnel: w325 -> [w363]
          tunnel: 2.0 -> [_]
          tunnel: w319 -> [w340]
          tunnel: 2.0 -> [w335]
          i -> [w348]
          stop <- w339 stop-if-true
          n151 = call "ADIS16448_RoboRIO_Teensy_GetData.vi"("SerialPortRefIn"=w362, "error in"=w366) -> ("IMU Angles Out"=w365:T12)  [unwired: 9 in, 4 out]
          n152 = Unbundle By Name(w365) -> ("Z Angle"=w345:dbl)
          n153 = Tick Count (ms)() -> (millisecond timer value=w343:u32)
          n154 = Equal To 0?(x=w348) -> (x = 0?=w357:bool)
          n155 = global read "Robot Global Data.vi" "Drive Select"() -> (w361:enum16{"WPI", "Platypi"})
          n156 = Subtract(x=w343, y=w340) -> (x-y=w342:u32)
          n157 = call "PIDF.vi"("reinitialize? (F)"=w357, "PIDF gains"="Rotate PID gains", "output range"="Rotate outputs", "process variable"=w345, "setpoint"=w346) -> ("output"=w355:dbl)  [unwired: 4 in, 2 out]
          n158 = Bundle(w346, "Z Angle"=w345) -> (→"Rotate Chart":cluster{dbl, "Z Angle":dbl})  [unwired: 1 in]
          n159 = Subtract(x=w346, y=w345) -> (x-y=→"RotateError":dbl)
          n160 = Absolute Value(x=w355) -> (abs(x)=w354:dbl)
          n161 = Divide(x=w342, y=u32 1000) -> (x/y=w336:dbl)
          n162 = Negate(x=w355) -> (-x=w360:dbl)
          n163 = case shown="\"WPI\", Default" w361 {
            tunnel: w364 -> [w371 w376]
            tunnel: w360 -> [w369 w373]
            tunnel: w363 -> [w368 w375]
            tunnel: w345 -> [w367 w372]
            frame "WPI", Default {
              w370 = 0.0 ("Y")
              # "Uses the WPI Drive VI"
              n164 = call-poly <vilib>:"WPI_RobotDriveHolonomicDrive.vi"("Rotation"=w369, "Gyro Angle"=w367, "error in (no error)"=w368, "Y"=w370, "X"=w370, "RobotDriveDevRef"=w371) -> ()  [unwired: 3 in, 3 out]
            }
            frame "Platypi" {
              w374 = 0.0 ("X")
              # "Uses the Platypi Drive VI"
              n165 = call "RobotDriveMecanumSRXSpeedControl_Cartesian.vi"("Rotation"=w373, "Gyro Angle"=w372, "error in (no error)"=w375, "Y"=w374, "X"=w374, "RobotDriveDevRef"=w376) -> ()  [unwired: 2 in, 4 out]
            }
          }
          n166 = Greater Or Equal?(x=w336, y=w335) -> (x >= y?=w337:bool)
          n167 = call <vilib>:"Mean PtByPt.vi"("x"=w354, "sample length"="RotateSampleLength") -> ("mean"=w352:dbl)  [unwired: 2 in, 1 out]
          n168 = Less?(x=w352, y="ExitLimitRotate") -> (x < y?=w350:bool)
          n169 = Greater?(x=w348, y="RotateIterationDelay") -> (0:w349:bool)
          n170 = And(x=w350, y=w349) -> (x .and. y?=w338:bool)
          n171 = Or(x=w338, y=w337) -> (x .or. y?=w339:bool)
        }
      }
      frame "VISION_ALIGN_ROTATE" {
        (unwired) 0.0
        # "Check for Invalid Data"
        # "If Vision Angle is +/- 1 deg from 0 (pointed at vision tape target)"
        # "Deg to rotate"
        # "Rotation Tolerance"
        # "Aligns the robot to the lifter to drop a gear."
        n172 = call "ADIS16448_RoboRIO_Teensy_GetData.vi"("SerialPortRefIn"=w397, "error in"=w396) -> ("SerialPortRefOut"=w389:T9, "IMU Angles Out"=w391:T12, "error out"=w388:errorcluster)  [unwired: 9 in, 2 out]
        n173 = global read "Robot Global Data.vi" "VisionAngle"() -> (w377:dbl)
        n174 = Unbundle By Name(w391) -> ("Z Angle"=w390:dbl)
        n175 = Equal?(x=w377, y=inf) -> (x = y?=w385:bool)
        n176 = call "Four Motor Set Brake Coast.vi"("Brake / Coast Mode"=WPI_CANTalonSRX_BrakeOverride."Override to Brake", "error in (no error)"=w394, "RobotDriveDevRef in"=w395) -> ("error out"=w379:errorcluster, "RobotDriveDevRef out"=w380:T10)  [unwired: 7 in]
        n177 = call "InRangeOfTarget.vi"("Tolerance"=1.0 ("Tolerence"), "Target"=0.0 ("y"), "Value"=w377) -> ("Is In Range"=w381:bool)
        n178 = Add(x=w390, y=w377) -> (x+y=w386:dbl)
        n179 = Or(x=w381, y=w385) -> (x .or. y?=w384:bool)
        n180 = case shown="False" w384 {
          tunnel: w380 -> [w403 _]
          tunnel: w379 -> [w402 _]
          tunnel: w386 -> [w401 _]
          tunnel: w389 -> [w400 _]
          tunnel: w388 -> [w399 _]
          frame False {
            n181 = Tick Count (ms)() -> (millisecond timer value=w398:u32)
            n182 = while {
              tunnel: w401 -> [w414]
              tunnel: w403 -> [w435]
              tunnel: w402 -> [w434]
              tunnel: w400 -> [w431]
              tunnel: w399 -> [w430]
              tunnel: w398 -> [w408]
              i -> [w417]
              stop <- w407 stop-if-true
              n183 = call "ADIS16448_RoboRIO_Teensy_GetData.vi"("SerialPortRefIn"=w431, "error in"=w430) -> ("IMU Angles Out"=w432:T12)  [unwired: 9 in, 4 out]
              n184 = Unbundle By Name(w432) -> ("Z Angle"=w413:dbl)
              n185 = Equal To 0?(x=w417) -> (x = 0?=w426:bool)
              n186 = Tick Count (ms)() -> (millisecond timer value=w411:u32)
              n187 = Bundle(w414, "Z Angle"=w413) -> (→"Vision Align Rotate Chart":cluster{dbl, "Z Angle":dbl})  [unwired: 1 in]
              n188 = call "PIDF.vi"("reinitialize? (F)"=w426, "PIDF gains"="Vision Align PID Gains", "output range"="Vision Align Limits", "process variable"=w413, "setpoint"=w414) -> ("output"=w415:dbl)  [unwired: 4 in, 2 out]
              n189 = global read "Robot Global Data.vi" "Drive Select"() -> (w433:enum16{"WPI", "Platypi"})
              n190 = Subtract(x=w411, y=w408) -> (x-y=w410:u32)
              n191 = Negate(x=w415) -> (-x=w425:dbl)
              n192 = case shown="\"Platypi\"" w433 {
                tunnel: w435 -> [w439 w443]
                tunnel: w425 -> [w437 w440]
                tunnel: w434 -> [w436 w442]
                frame "WPI", Default {
                  w438 = 0.0 ("Y")
                  # "Uses the WPI Drive VI"
                  n193 = call-poly <vilib>:"WPI_RobotDriveHolonomicDrive.vi"("Rotation"=w437, "error in (no error)"=w436, "Y"=w438, "X"=w438, "RobotDriveDevRef"=w439) -> ()  [unwired: 4 in, 3 out]
                }
                frame "Platypi" {
                  w441 = 0.0 ("X")
                  # "Uses the Platypi Drive VI"
                  n194 = call "RobotDriveMecanumSRXSpeedControl_Cartesian.vi"("Rotation"=w440, "error in (no error)"=w442, "Y"=w441, "X"=w441, "RobotDriveDevRef"=w443) -> ()  [unwired: 3 in, 4 out]
                }
              }
              n195 = Divide(x=w410, y=u32 1000) -> (x/y=w405:dbl)
              n196 = Absolute Value(x=w415) -> (abs(x)=w424:dbl)
              n197 = Greater Or Equal?(x=w405, y=1.0 ("x")) -> (x >= y?=w406:bool)
              n198 = call <vilib>:"Mean PtByPt.vi"("x"=w424, "sample length"="VisionSampleLength") -> ("mean"=w416:dbl)  [unwired: 2 in, 1 out]
              n199 = Subtract(x=w414, y=w413) -> (x-y=→"VisionError":dbl)
              n200 = Less?(x=w416, y="ExitLimitVision") -> (x < y?=w421:bool)
              n201 = Greater?(x=w417, y="VisionIterationDelay") -> (0:w420:bool)
              n202 = And(x=w421, y=w420) -> (x .and. y?=w418:bool)
              n203 = Or(x=w418, y=w406) -> (x .or. y?=w407:bool)
            }
          }
          frame True {
          }
        }
      }
      frame "SHOOT_HIGH" {
        # "Initial time."
        # "Shoots fuel for x seconds while running the agitator."
        n204 = Tick Count (ms)() -> (millisecond timer value=w450:u32)
        n205 = while {
          tunnel: w450 -> [w459]
          tunnel: w445 -> [w458]
          tunnel: w449 -> [w453]
          tunnel: w448 -> [w452]
          tunnel: w447 -> [w456]
          tunnel: w446 -> [w455]
          stop <- w457 continue-if-true
          # "Takes the intital time and will continuously shoot until the allotted time has passed."
          # "Current time."
          n206 = call "ShooterMotorSpeedControl.vi"("error in"=w452, "Go?"=TRUE, "CAN Talon SRX Ref"=w453) -> ()  [unwired: 6 in, 3 out]
          n207 = Tick Count (ms)() -> (millisecond timer value=w463:u32)
          n208 = global read "Robot Global Data.vi" "Drive Select"() -> (w454:enum16{"WPI", "Platypi"})
          n209 = Subtract(x=w463, y=w459) -> (x-y=w462:u32)
          n210 = case shown="\"WPI\", Default" w454 {
            tunnel: w456 -> [w464 w470]
            tunnel: w455 -> [w465 w469]
            frame "WPI", Default {
              w466 = 0.0 ("Y")
              # "Uses the WPI Drive VI"
              n211 = call-poly <vilib>:"WPI_RobotDriveHolonomicDrive.vi"("Rotation"=w466, "error in (no error)"=w465, "Y"=w466, "X"=w466, "RobotDriveDevRef"=w464) -> ()  [unwired: 4 in, 3 out]
            }
            frame "Platypi" {
              w468 = 0.0 ("X")
              # "Uses the Platypi Drive VI"
              n212 = call "RobotDriveMecanumSRXSpeedControl_Cartesian.vi"("Rotation"=0.0, "error in (no error)"=w469, "Y"=w468, "X"=w468, "RobotDriveDevRef"=w470) -> ()  [unwired: 3 in, 4 out]
            }
          }
          n213 = Divide(x=w462, y=u32 1000) -> (x/y=w460:dbl)
          n214 = Greater Or Equal?(x=w458, y=w460) -> (x >= y?=w457:bool)
        }
      }
      frame "OPEN_GATE" {
        # "Opens the gate to drop a gear."
        n215 = call <vilib>:"WPI_ServoSetAngle.vi"("error in (no error)"=w476, "Angle"=170.0, "ServoDeviceRef"=w477) -> ()  [unwired: 7 in, 2 out]
        n216 = call <vilib>:"WPI_ServoSetAngle.vi"("error in (no error)"=w474, "Angle"=0, "ServoDeviceRef"=w475) -> ()  [unwired: 7 in, 2 out]
      }
      frame "CLOSE_GATE" {
        # "Closes the gate to hold a gear."
        n217 = call <vilib>:"WPI_ServoSetAngle.vi"("error in (no error)"=w484, "Angle"=0.0, "ServoDeviceRef"=w485) -> ()  [unwired: 7 in, 2 out]
        n218 = call <vilib>:"WPI_ServoSetAngle.vi"("error in (no error)"=w482, "Angle"=170, "ServoDeviceRef"=w483) -> ()  [unwired: 7 in, 2 out]
      }
    }
    n219 = call-poly <vilib>:"NT Write Value.vi"("Numeric"=w24, "Name"="ArgOutput") -> ()  [unwired: 9 in, 1 out]
    n220 = call-poly <vilib>:"NT Write Value.vi"("String"=w25, "Name"="AutoOutput") -> ()  [unwired: 9 in, 1 out]
  }
